vi "WaitV2.vi"(8 "error in (no error)":errorcluster, 11 "ChirpV2 in":refnum<class "ChirpV2.lvclass">) -> (0 "error out":errorcluster, 2 "data":dynamicdata(graph), 3 "ChirpV2 out":refnum<class "ChirpV2.lvclass">)   [LabVIEW 2014, in "ChirpV2.lvclass"]
uses:
  ChirpV2.lvclass
  <vilib>/measure/NI_MABase.lvlib
  <vilib>/addons/_NISVFA/_Generation/SoundVib_Generation.lvlib
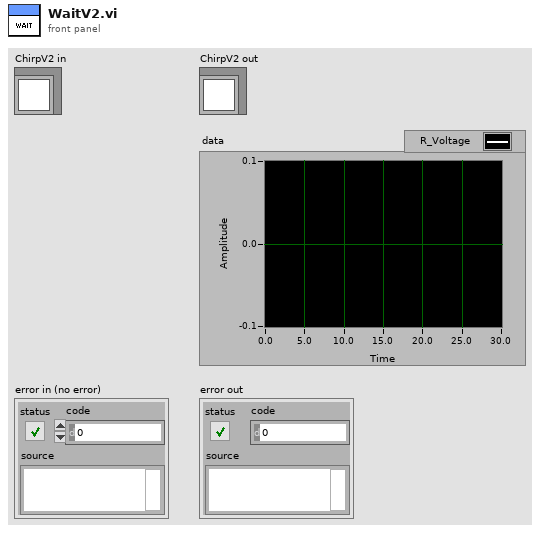
[diagram p1: front panel]
types:
  T1 = cluster{"start frequency [Hz]":dbl, "stop frequency [Hz]":dbl}
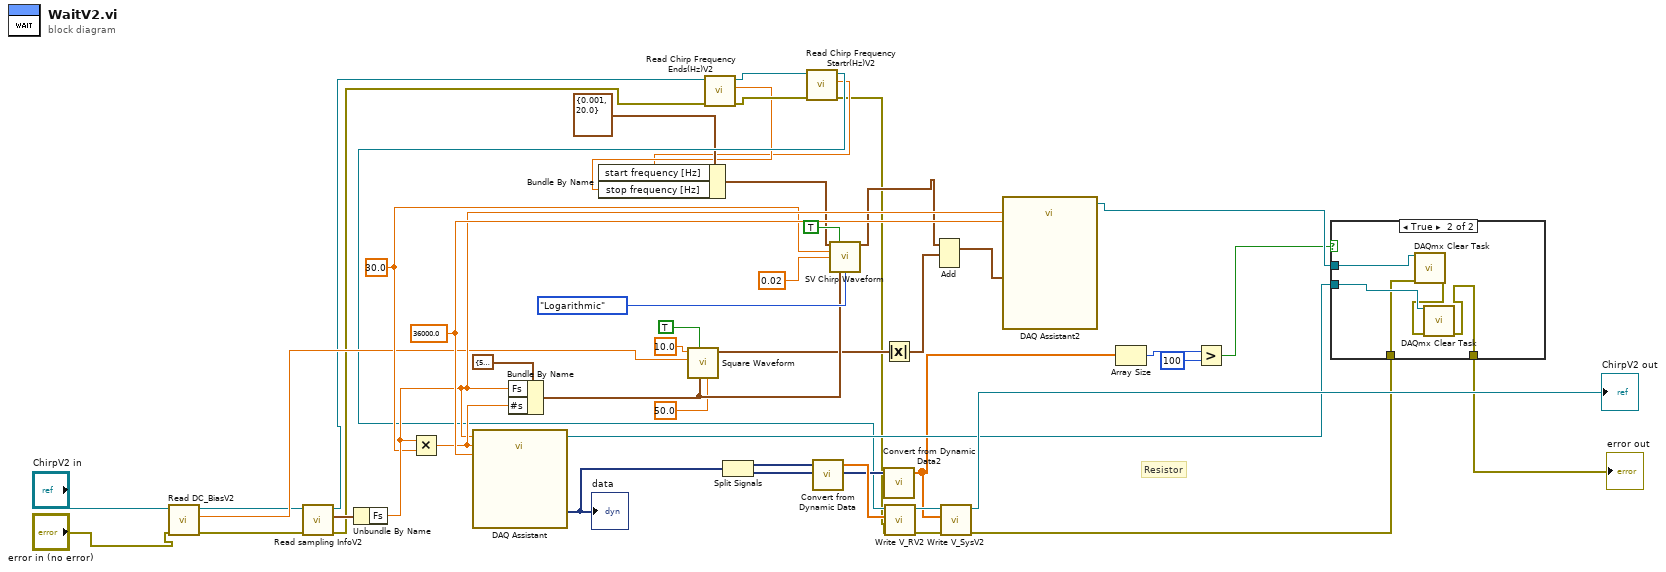
[diagram p0: block diagram]
diagram:
  w40 = 36000.0 ("timeout (s)")
  w35 = 30.0 ("y")
  # "Resistor"
  n1 = call-dynamic "Read DC_BiasV2.vi"("error in (no error)"="error in (no error)", "ChirpV2 in"="ChirpV2 in") -> ("error out"=w27:errorcluster, "DC_Bias"=w28:dbl, "ChirpV2 out"=w26:refnum<class "ChirpV2.lvclass">)  [unwired: 7 in]
  n2 = call-dynamic "Read sampling InfoV2.vi"("error in (no error)"=w27, "ChirpV2 in"=w26) -> ("error out"=w2:errorcluster, "sampling Info"=w29:cluster{"Fs":dbl}, "ChirpV2 out"=w8:refnum<class "ChirpV2.lvclass">)  [unwired: 7 in]
  n3 = Unbundle By Name(w29) -> ("Fs"=w38:dbl)
  n4 = Multiply(x=w38, y=w35) -> (x*y=w39:dbl)
  n5 = call "DAQ Assistant"("rate"=w38, "number of samples"=w39, "timeout (s)"=w40) -> ("task out"=w18:refnum<k21>, "data"=w43:dynamicdata)  [unwired: 14 in, 1 out]
  "data" <- w43
  n6 = Bundle By Name(cluster=cluster{"Fs":dbl, "#s":u32} {"Fs"=51200.0, "#s"=1024} ("sampling info"), "Fs"=w38, "#s"=w39) -> (w31:cluster{"Fs":dbl, "#s":u32})
  n7 = call <vilib>:"Square Waveform.vi"("duty cycle (%)"=50.0, "sampling info"=w31, "reset signal"=TRUE, "amplitude"=w28, "frequency"=10.0) -> ("signal out"=w24:waveform(dbl))  [unwired: 5 in, 1 out]
  n8 = call-dynamic "Read Chirp Frequency Ends(Hz)V2.vi"("error in (no error)"=w2, "ChirpV2 in"=w8) -> ("error out"=w9:errorcluster, "Chirp Frequency Ends(Hz)"=w4:dbl, "ChirpV2 out"=w10:refnum<class "ChirpV2.lvclass">)  [unwired: 7 in]
  n9 = Split Signals(w43) -> (w41:dynamicdata, w42:dynamicdata)  [unwired: 2 in]
  n10 = call-dynamic "Read Chirp Frequency Startr(Hz)V2.vi"("error in (no error)"=w9, "ChirpV2 in"=w10) -> ("error out"=w1:errorcluster, "Chirp Frequency Startr(Hz)"=w3:dbl, "ChirpV2 out"=w7:refnum<class "ChirpV2.lvclass">)  [unwired: 7 in]
  n11 = Bundle By Name(cluster=T1 {"start frequency [Hz]"=0.001, "stop frequency [Hz]"=20.0} ("frequency range"), "start frequency [Hz]"=w3, "stop frequency [Hz]"=w4) -> (w5:T1)
  n12 = call "Convert from Dynamic Data"("Dynamic Data Type"=w41) -> ("Array"=w44:dbl[])  [unwired: 3 in]
  n13 = call <vilib>:"SV Chirp Waveform.vi"("frequency range"=w5, "reset signal (F)"=TRUE, "chirp duration [s]"=w35, "amplitude"=0.02, "sampling info"=w31, "frequency spacing"=enum16{"Linear", "Logarithmic"}."Logarithmic") -> ("chirp signal"=w11:waveform(dbl))  [unwired: 7 in, 2 out]
  n14 = Absolute Value(x=w24) -> (abs(x)=w33:waveform(dbl))
  n15 = call "Convert from Dynamic Data2"("Dynamic Data Type"=w42) -> ("Array"=w17:dbl[])  [unwired: 3 in]
  n16 = call-dynamic "Write V_RV2.vi"("error in (no error)"=w1, "V_R"=w44, "ChirpV2 in"=w7) -> ("error out"=w46:errorcluster, "ChirpV2 out"=w45:refnum<class "ChirpV2.lvclass">)  [unwired: 7 in]
  n17 = Add(1:w33, 2:w11) -> (0:w34:waveform(dbl))  [unwired: 1 in, 1 out]
  n18 = call-dynamic "Write V_SysV2.vi"("error in (no error)"=w46, "V_Sys"=w17, "ChirpV2 in"=w45) -> ("error out"=w13:errorcluster, "ChirpV2 out"=→"ChirpV2 out":refnum<class "ChirpV2.lvclass">)  [unwired: 7 in]
  n19 = call "DAQ Assistant2"("data"=w34, "rate"=w38, "timeout (s)"=w40) -> ("task out"=w19:refnum<k21>)  [unwired: 14 in, 2 out]
  n20 = Array Size(array=w17) -> (size(s)=w16:i32)
  n21 = Greater?(x=w16, y=100) -> (0:w15:bool)
  n22 = case shown="True" w15 {
    tunnel: w18 -> [_ w52]
    tunnel: w19 -> [_ w53]
    tunnel: w13 -> [w48 w51]
    tunnel: [w48 w49] -> w12
    frame False {
    }
    frame True {
      n23 = call <vilib>:"DAQmx Clear Task.vi"("task in"=w53, "error in"=w51) -> ("error out"=w50:errorcluster)  [unwired: 13 in]
      n24 = call <vilib>:"DAQmx Clear Task.vi"("task in"=w52, "error in"=w50) -> ("error out"=w49:errorcluster)  [unwired: 13 in]
    }
  }
  "error out" <- w12
